vi "GetLOT.vi"(8 "错误输入":errorcluster) -> (0 "错误输出":errorcluster, 2 "生产批次有效":bool, 3 "LOT":string)   [LabVIEW 2020]
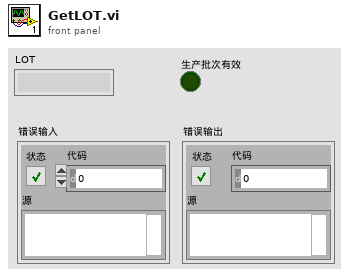
[diagram p1: front panel]
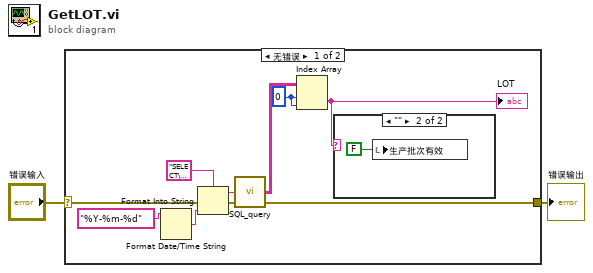
[diagram p0: block diagram]
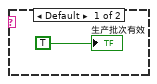
[diagram p2: hidden frame]
diagram:
  n1 = case shown="无错误" "错误输入" {
    selector: "错误输入" -> [w7 w15]
    tunnel: [w5 w15] -> w1
    frame No Error {
      w8 = 0 ("索引 (行)")
      n2 = Format Date/Time String(time format string (%c)="%Y-%m-%d" ("时间格式字符串(%c)")) -> (date/time string=w10:string)  [unwired: 2 in]
      n3 = Format Into String(format string="SELECT\ndbo.[生产计划].[生产编号]\n\nFROM\ndbo.[生产计划]\nWHERE\ndbo.[生产计划].[日期] = '%s' AND\ndbo.[生产计划].[计划状态] = '已审核'", error in=w7, w10) -> (resulting string=w9:string, error out=w6:errorcluster)  [unwired: 1 in]
      n4 = call "SQL_query.vi"("error in (no error)"=w6, "SQL query"=w9) -> ("error out"=w5:errorcluster, "data"=w4:string[][])  [unwired: 1 in, 1 out]
      n5 = Index Array(array=w4, index (row)=w8, index (col)=w8) -> (element=w3:string)
      "LOT" <- w3
      n6 = case shown="\"\"" w3 {
        frame Default {
          "生产批次有效" <- TRUE
        }
        frame "" {
          n7 = local write "生产批次有效"(FALSE ("生产批次有效")) -> ()
        }
      }
    }
    frame Error {
    }
  }
  "错误输出" <- w1
